vi "Get Internal Data Info.vi"(8 "error in (no error)":errorcluster, 11 "CSM-Helper in":refnum<class "CSM-Helper.lvclass">) -> (0 "error out":errorcluster, 2 "Array":T1[](array[typedef]), 3 "CSM-Helper out":refnum<class "CSM-Helper.lvclass">)   [LabVIEW 2017, in "CSM-Helper.lvclass"]
doc: "### Get Internal Data Info.vi\n\n-- <b>Controls</b> --\n- <b>CSM-Helper in</b>: CSMHelper input\n\n-- <b>Indicators</b> --\n- <b>Array</b>:\n- <b>CSM-Helper out</b>: CSMHelper output"
uses:
  CSM-Helper.lvclass
  Typedef/Def-Internal Data Info.ctl
  CSM-Helper.lvclass/CSM-Helper.ctl
  <vilib>/Utility/Data Type/NI_Data Type.lvlib
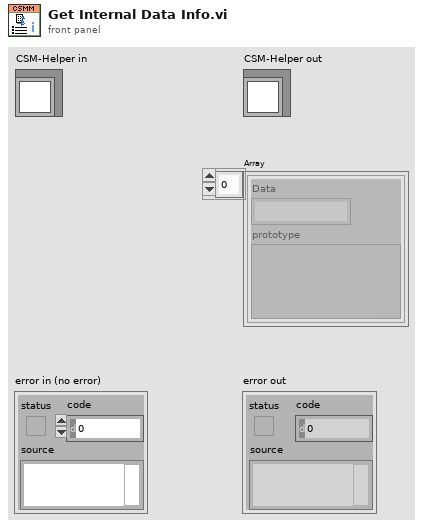
[diagram p1: front panel]
types:
  T1 = typedef "CSM-Helper.lvclass/Def-Internal Data Info.ctl" = cluster{"Data":string, "prototype":variant}
  T2 = typedef "NI_Data Type.lvlib/Data Type.ctl" = enum8{"Invalid Type", "Void", "I8", "I16", "I32", "I64", "U8", "U16", "U32", "U64", "Single Float", "Double Float", "Extended Float", "Single Complex", "Double Complex", "Extended Complex", "Enum U8", "Enum U16", "Enum U32", "Enum U64", "Single Float With Unit", "Double Float With Unit", "Extended Float With Unit", "Single Complex with Unit", "Double Complex with Unit", "Extended Complex with Unit", "Boolean", "String", "Path", "Picture", "Tag", "Array", "Cluster", "Variant", "LV Variant", "Waveform", "Timestamp", "Digital Waveform", "Digital Data", "ExpressData", "Refnum", "External Data", "VI", "Poly VI", "LabVIEW Class Instance", "Fixed Point"}
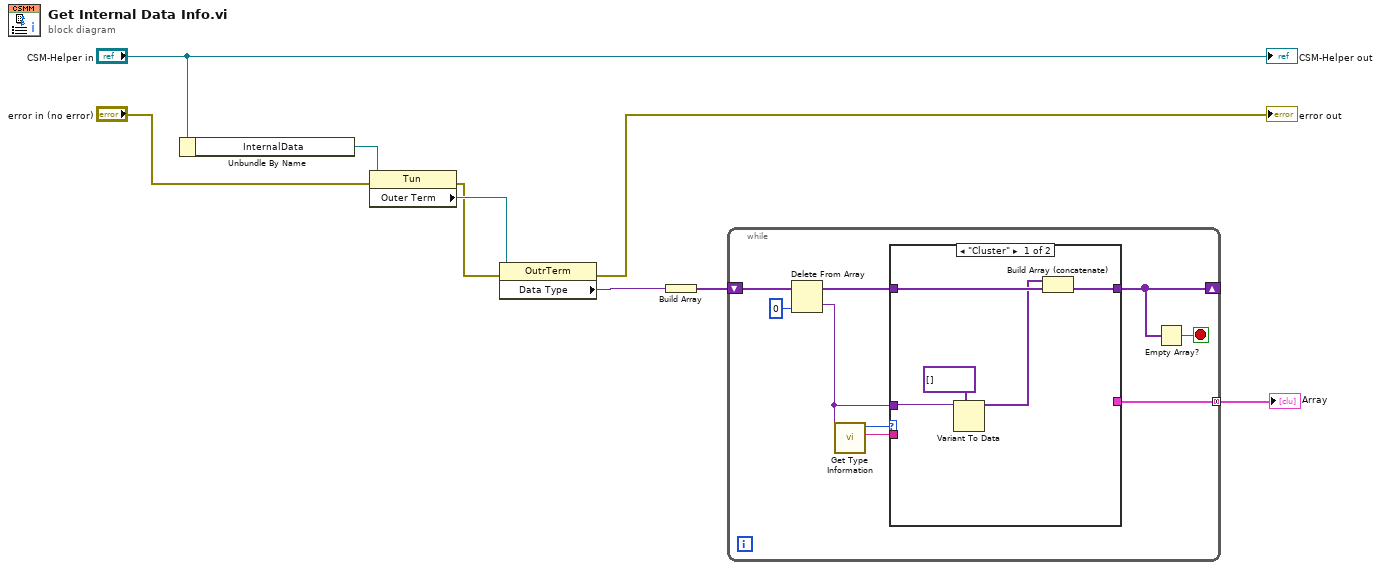
[diagram p0: block diagram]
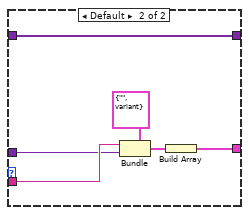
[diagram p2: hidden frame]
diagram:
  n1 = Unbundle By Name("CSM-Helper in") -> ("InternalData"=w8:refnum<vi>)
  n2 = property class="Tun"(reference=w8, error in="error in (no error)") -> (error out=w5:errorcluster, "Outer Term"=w7:refnum<vi>)  [unwired: 1 out]
  n3 = property class="OutrTerm"(reference=w7, error in=w5) -> (error out=→"error out":errorcluster, "Data Type"=w2:variant)  [unwired: 1 out]
  n4 = Build Array(w2) -> (w1:variant[])
  n5 = while {
    tunnel: [w14] -> w6 mode=concatenating
    shift-right: [w10] -> _
    shift-left: w1 -> [w18]
    stop <- w11 stop-if-true
    n6 = Delete From Array(array=w18, index=0) -> (deleted portion=w15:variant, array with subset deleted=w12:variant[])  [unwired: 1 in]
    n7 = call <vilib>:"Get Type Information.vi"("Variant"=w15) -> ("Name"=w16:string, "Type"=w13:T2)  [unwired: 6 in, 3 out]
    n8 = case shown="\"Cluster\"" w13 {
      tunnel: w16 -> [_ w28]
      tunnel: w15 -> [w22 w27]
      tunnel: [_ w25] -> w14
      tunnel: w12 -> [w21 w24]
      tunnel: [w20 w24] -> w10
      frame "Cluster" {
        n9 = Variant To Data(type=variant[] [] ("Array"), Variant=w22) -> (data=w19:variant[])  [unwired: 1 in, 1 out]
        n10 = Build Array (concatenate)(w19, w21) -> (w20:variant[])
      }
      frame Default {
        n11 = Bundle(cluster=T1 {"Data"="", "prototype"=variant}, "Data"=w28, "prototype"=w27) -> (w29:T1)
        n12 = Build Array(w29) -> (w25:T1[])
      }
    }
    n13 = Empty Array?(array=w10) -> (empty?=w11:bool)
  }
  "Array" <- w6
  "CSM-Helper out" <- "CSM-Helper in"
